vi "Wait for Exit.vi"(6 "deadline":T1={"mode"=enum."Relative", "deadline (ms)"=30000}, 8 "error in (no error)":errorcluster, 11 "subprocess in":refnum<class "Buffered Subprocess.lvclass">) -> (0 "error out":errorcluster, 2 "return code":u8, 3 "subprocess out":refnum<class "Buffered Subprocess.lvclass">)   [LabVIEW 2020, in "NI_Subprocess.lvlib" / "Buffered Subprocess.lvclass"]
uses:
  <vilib>/Subprocess/Buffered Subprocess/Buffered Subprocess.lvclass
  <vilib>/Utility/Deadline/Deadline.ctl
  <vilib>/Utility/Deadline/Mode.ctl
  <vilib>/Subprocess/Buffered Subprocess/Buffered Subprocess.lvclass/Buffered Subprocess.ctl
  <vilib>/Subprocess/Subprocess/Subprocess.lvclass
  <vilib>/Utility/Deadline/NI_Deadline.lvlib
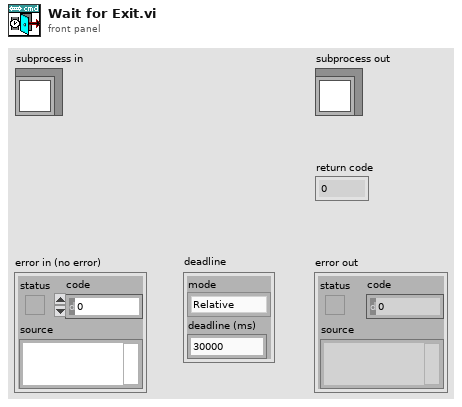
[diagram p1: front panel]
types:
  T1 = typedef "NI_Deadline.lvlib/Deadline.ctl" = cluster{"mode":T2, "deadline (ms)":u32}
  T2 = typedef "NI_Deadline.lvlib/Mode.ctl" = enum16{"Relative", "Use deadline", "Wait forever", "Nonblocking", "N/A"}
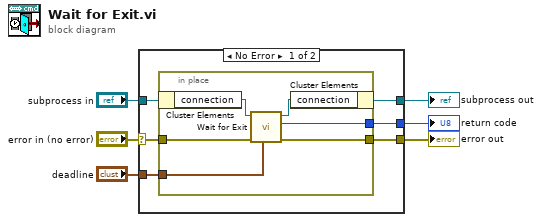
[diagram p0: block diagram]
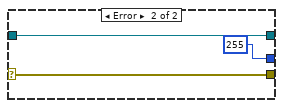
[diagram p2: hidden frame]
diagram:
  n1 = case shown="No Error" "error in (no error)" {
    selector: "error in (no error)" -> [w11 w21]
    tunnel: [w10 w21] -> w5
    tunnel: [w8 w20] -> w3
    tunnel: "subprocess in" -> [w12 w20]
    tunnel: [w9 u8 255 ("return code")] -> w2
    tunnel: "deadline" -> [w7 _]
    frame No Error {
      n2 = in-place {
        in-place-border: w11 -> [w16]
        in-place-border: [w15] -> w10
        in-place-border: [w14] -> w9
        in-place-border: w7 -> [w13]
        n3 = in-place-cluster #1(w12) -> ("connection"=w18:refnum<class "Subprocess.lvclass">)
        n4 = call <vilib>:"Wait for Exit.vi"("deadline"=w13, "error in (no error)"=w16, "subprocess in"=w18) -> ("error out"=w15:errorcluster, "return code"=w14:u8, "subprocess out"=w17:refnum<class "Subprocess.lvclass">)  [unwired: 6 in]
        n5 = in-place-cluster #1("connection"=w17) -> (w8:refnum<class "Buffered Subprocess.lvclass">)
      }
    }
    frame Error {
    }
  }
  "error out" <- w5
  "subprocess out" <- w3
  "return code" <- w2
